vi "CreateDriveTrain.vi"   [LabVIEW 2016]
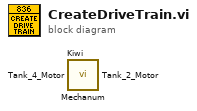
[diagram p0: block diagram]
diagram:
  n1 = call <userlib>:"Mechanum.vi"() -> ()  [unwired: 12 in]
  n2 = call <userlib>:"Kiwi.vi"() -> ()  [unwired: 12 in]
  n3 = call <userlib>:"Tank_4_Motor.vi"() -> ()  [unwired: 11 in, 1 out]
  n4 = call <userlib>:"Tank_2_Motor.vi"() -> ()  [unwired: 11 in, 1 out]
